vi "Pockels modulation-Gen AO seq for non-funct img.vi"(9 "Imaging Protocol":T1, 11 "Setup/Logging queue element":T2={"Imaging Protocol"=enum."Live Imaging", "Number of Trials"=0, "Frame Size"=512, "# Averaged frames"=0, "Dwell time (us)"=0.0, "Index of Z-plane"=0, "Timelapse?"=FALSE, "Logging process is active"=FALSE, "Speed logging enabled"=FALSE, "tdms file ref"=refnum, "path"=path "", "Trial Number"=0, "Expected # points acquired"=FALSE, "Manually stopped"=FALSE, "Last trial"=FALSE, "Ch0 data"=[], "Ch1 data"=[], "Image Time"=[], "Continuous Time"=[], "Points acquired"={"Ch0 last trial"=0, "Ch1 last trial"=0, "All trials"=0}, "HW Timings File"=refnum} {"Frame Size" items=["100X100"=100, "128X128"=128, "200X200"=200, "256X256"=256, "512X512"=512, "1024x1024"=1024, "2048x2048"=2048]; "Dwell time (us)" format="%#.6g"}) -> (1 "Pockels modulation AO sequence":dbl[](array[numeric]), 2 "Sampling period (us)":dbl format="%#_6f", 3 "Length of sequence (ms)":dbl format="%#_6f", 4 "Data length (points)":i32)   [LabVIEW 2017]
uses:
  Typedefs/Logging queue element.ctl
  Typedefs/Imaging Protocols enum.ctl
  Typedefs/Frame Size.ctl
  Typedefs/Acquired points count.ctl
  Typedefs/Pockels mod gen variables cluster.ctl
  Globals/gl_Pockels control globals.vi
  Global Variables/General Globals.vi
panel:
  out "Pockels modulation waveform":dbl[](graph)
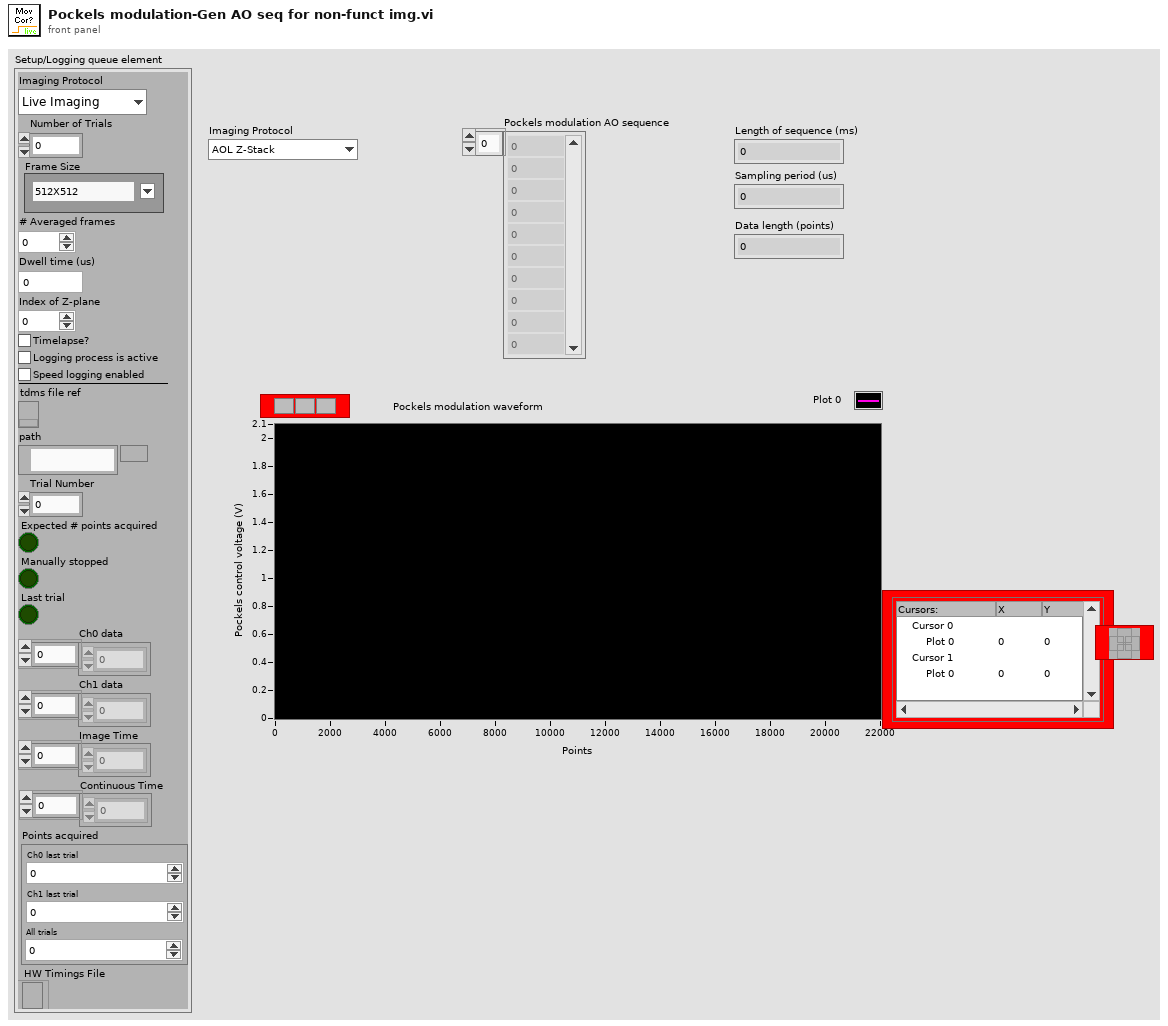
[diagram p1: front panel]
types:
  T1 = typedef "Imaging Protocols enum.ctl" = enum16{"AOL Z-Stack", "Motor Z Stack", "Functional Acquisition", "Single Plane Acquisition", "Volume Acquisition", "Live Imaging", "Live Plane Imaging", "Live Volume Imaging"}
  T2 = typedef "Logging queue element.ctl" = cluster{"Imaging Protocol":T1, "Number of Trials":u16, "Frame Size":T3, "# Averaged frames":u16, "Dwell time (us)":dbl, "Index of Z-plane":i32, "Timelapse?":bool, "Logging process is active":bool, "Speed logging enabled":bool, "tdms file ref":refnum<k34>, "path":path, "Trial Number":i32, "Expected # points acquired":bool, "Manually stopped":bool, "Last trial":bool, "Ch0 data":u32[], "Ch1 data":u32[], "Image Time":u64[], "Continuous Time":u64[], "Points acquired":T4, "HW Timings File":refnum<file>}
  T3 = typedef "Frame Size.ctl" = u16
  T4 = typedef "Acquired points count.ctl" = cluster{"Ch0 last trial":u64, "Ch1 last trial":u64, "All trials":u64}
  T5 = typedef "Pockels mod gen variables cluster.ctl" = cluster{"Dwell time":dbl, "Number of frame lines":i32, "Number of points in a line":i32, "Index of Z-plane":i32, "Pockels \"Low\" time (us)":dbl, "Sample Clock Rate":dbl, "Imaging Protocol":T1}
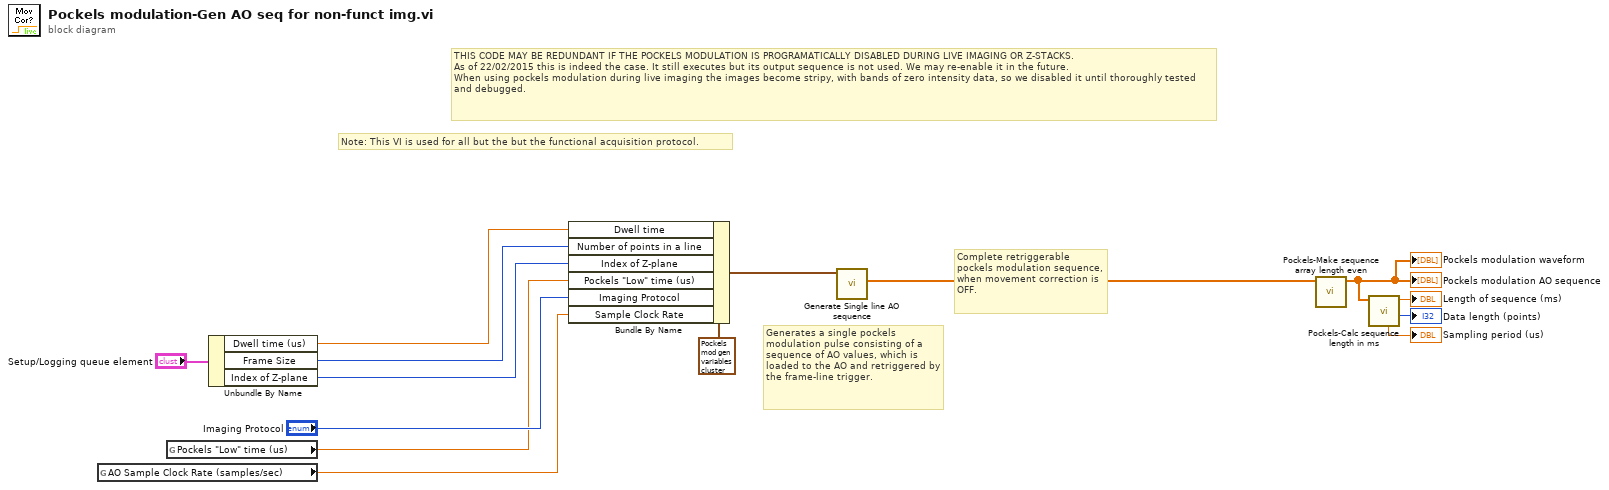
[diagram p0: block diagram]
diagram:
  # "Complete retriggerable pockels modulation sequence, when movement correction is OFF."
  # "Generates a single pockels modulation pulse consisting of a sequence of AO values, which is loaded to the AO and retriggered by the frame-line trigger."
  # "THIS CODE MAY BE REDUNDANT IF THE POCKELS MODULATION IS PROGRAMATICALLY DISABLED DURING LIVE IMAGING OR Z-STACKS.\nAs of 22/02/2015 this is indeed the case. It still executes but its output sequence is not used. We may re-enable it in the future.\nWhen using pockels modulation during live imaging the images become stripy, with bands of zero intensity data, so we disabled it until thoroughly tested and debugged."
  # "Note: This VI is used for all but the but the functional acquisition protocol."
  n1 = global read "General Globals.vi" "AO Sample Clock Rate (samples/sec)"() -> (w7:dbl)
  n2 = global read "gl_Pockels control globals.vi" "Pockels \"Low\" time (us)"() -> (w10:dbl)
  n3 = Unbundle By Name("Setup/Logging queue element") -> ("Dwell time (us)"=w11:dbl, "Frame Size"=w12:T3, "Index of Z-plane"=w13:i32)
  n4 = Bundle By Name(cluster=T5 {"Dwell time"=0.0, "Number of frame lines"=512, "Number of points in a line"=0, "Index of Z-plane"=0, "Pockels \"Low\" time (us)"=0.0, "Sample Clock Rate"=0.0, "Imaging Protocol"=enum."AOL Z-Stack"} ("Variables"), "Dwell time"=w11, "Number of points in a line"=w12, "Index of Z-plane"=w13, "Pockels \"Low\" time (us)"=w10, "Imaging Protocol"="Imaging Protocol", "Sample Clock Rate"=w7) -> (w2:T5)
  n5 = call "Generate Single line AO sequence.vi"("Variables"=w2) -> ("Single line AO sequence"=w8:dbl[])  [unwired: 10 in]
  n6 = call "Pockels-Make sequence array length even.vi"("Single line AO sequence in"=w8) -> ("Single line AO sequence out"=w6:dbl[])  [unwired: 10 in]
  "Pockels modulation AO sequence" <- w6
  "Pockels modulation waveform" <- w6
  n7 = call "Pockels-Calc sequence length in ms.vi"("Pockels modulation sequence in"=w6) -> ("Sequence length (points)"=→"Data length (points)":i32, "Sequence length (ms)"=→"Length of sequence (ms)":dbl, "Sampling period (us)"=→"Sampling period (us)":dbl)  [unwired: 8 in]
